vi "Ex3_Serial_Write_Read.vi"(0 "VISA resource":refnum<visa-resource-name>="COM4", 5 "Comando":T2(ring), 7 "Decisión":bool, 9 "stop":bool, 11 "error in (no error)":errorcluster) -> (3 "VISA resource 2":refnum<visa-resource-name>="COM4", 4 "Señales Digitales":dynamicdata(graph), 6 "Señales Analógicas":dynamicdata(graph), 8 "Buffer Filtrado":string, 10 "Cluster Señales":T1, 15 "error out":errorcluster)   [LabVIEW 2020]
uses:
  <vilib>/Instr/_visa.llb/VISA Configure Serial Port (Instr).vi
panel:
  out "Buffer Completo":string
  out "LISTO?":bool=TRUE
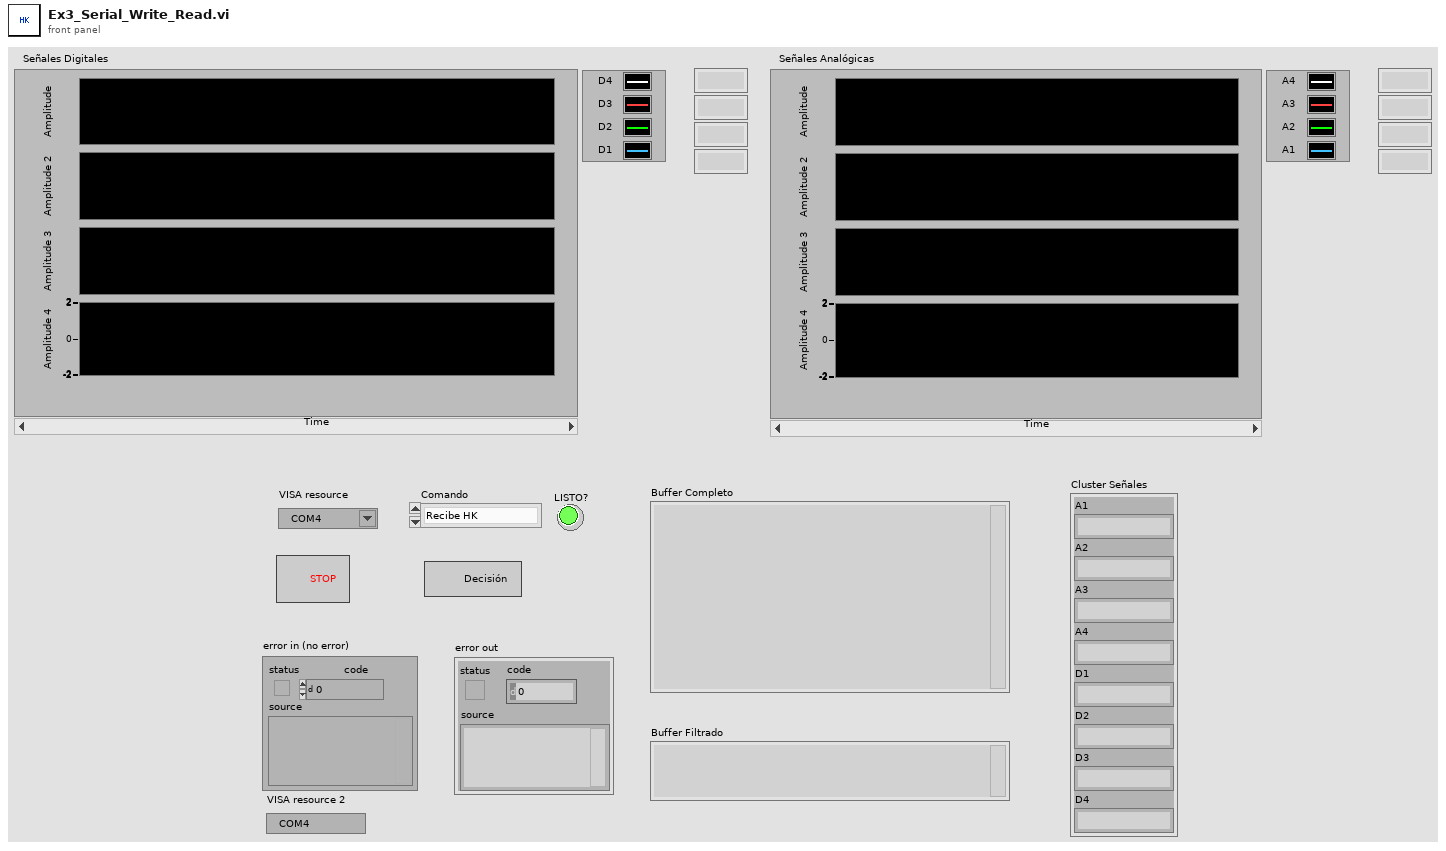
[diagram p1: front panel]
types:
  T1 = cluster{"A1":string, "A2":string, "A3":string, "A4":string, "D1":string, "D2":string, "D3":string, "D4":string}
  T2 = enum16{"Recibe HK", "Act Fecha", "Parametros", "Reset", "Stop"}
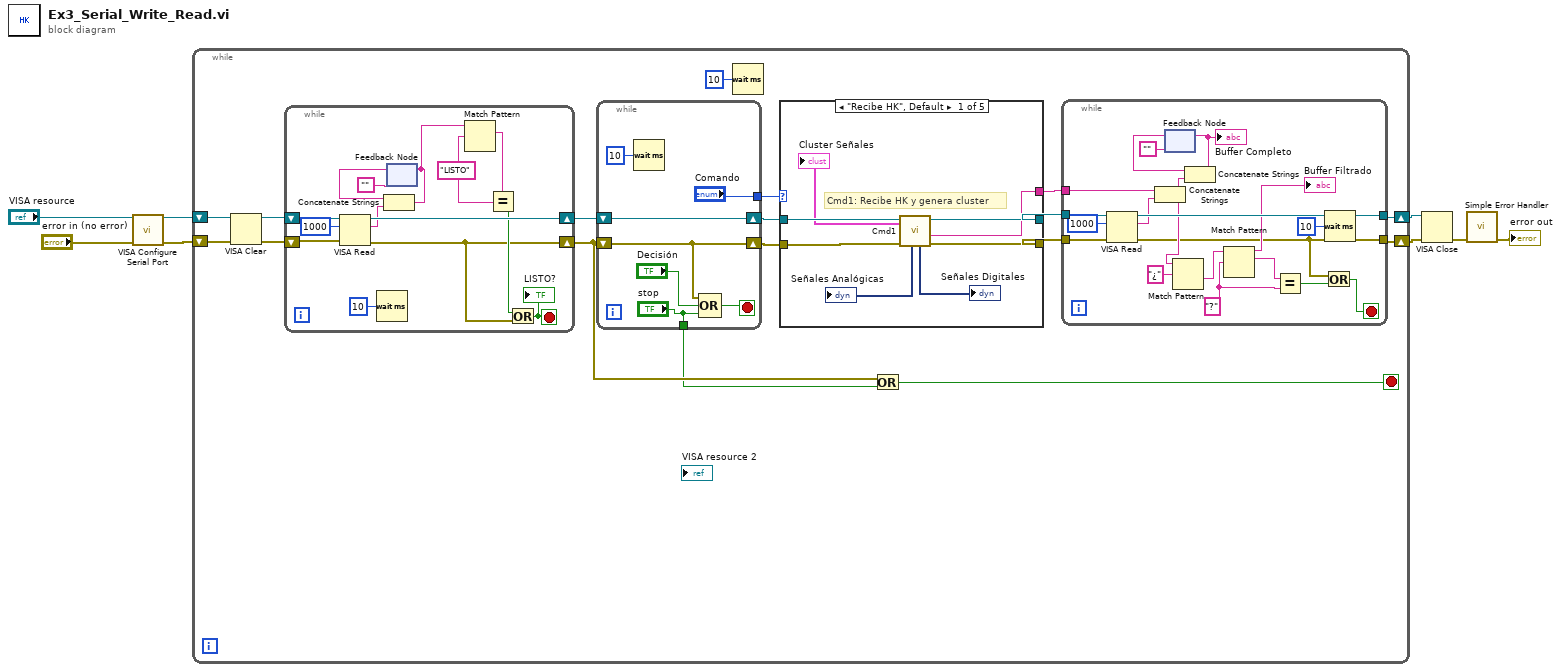
[diagram p0: block diagram]
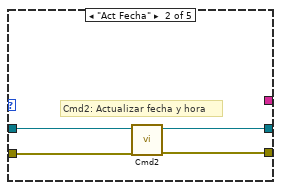
[diagram p2: hidden frame]
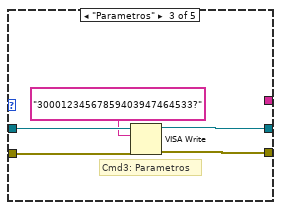
[diagram p3: hidden frame]
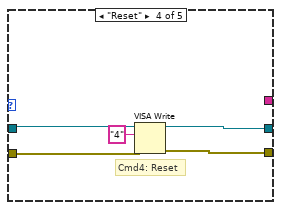
[diagram p4: hidden frame]
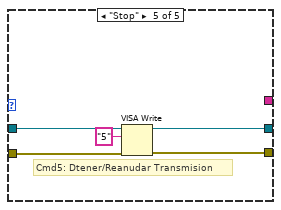
[diagram p5: hidden frame]
diagram:
  n1 = call-poly "VISA Configure Serial Port"("VISA resource name"="VISA resource", "error in (no error)"="error in (no error)") -> ("VISA resource name out"=w2:refnum<visa-resource-name>, "error out"=w1:errorcluster)  [unwired: 12 in]
  n2 = while {
    shift-right: [w12] -> w5
    shift-left: w1 -> [w18]
    shift-right: [w13] -> w6
    shift-left: w2 -> [w20]
    stop <- w21 stop-if-true
    n3 = VISA Clear(VISA resource name=w20, error in (no error)=w18) -> (VISA resource name out=w19:refnum<visa-resource-name>, error out=w17:errorcluster)
    n4 = while {
      shift-right: [w80] -> w11
      shift-left: w17 -> [w91]
      shift-right: [w89] -> w23
      shift-left: w19 -> [w92]
      stop <- w79 stop-if-true
      w82 = "LISTO" ("regular expression")
      n5 = VISA Read(VISA resource name=w92, byte count=u32 1000, error in (no error)=w91) -> (VISA resource name out=w89:refnum<visa-resource-name>, read buffer=w88:string, error out=w80:errorcluster)  [unwired: 1 out]
      n6 = Wait (ms)(milliseconds to wait=u32 10) -> ()  [unwired: 1 out]
      n7 = feedback #1("") -> (w87:string)
      n8 = Concatenate Strings(w87, w88) -> (w84:string)
      n9 = feedback-in #1(w84) -> ()
      n10 = Match Pattern(string=w84, regular expression=w82) -> (match substring=w83:string)  [unwired: 1 in, 3 out]
      n11 = Equal?(x=w83, y=w82) -> (x = y?=w81:bool)
      n12 = Or(x=w81, y=w80) -> (x .or. y?=w79:bool)
      "LISTO?" <- w79
    }
    n13 = while {
      tunnel: ["Comando"] -> w25
      shift-right: [w50] -> w24
      shift-left: w23 -> [w50]
      shift-right: [w47] -> w22
      shift-left: w11 -> [w47]
      tunnel: ["stop"] -> w10
      stop <- w48 stop-if-true
      n14 = Wait (ms)(milliseconds to wait=u32 10) -> ()  [unwired: 1 out]
      n15 = Compound Arithmetic op=OR(w47, "Decisión", "stop") -> (w48:bool)
    }
    n16 = Wait (ms)(milliseconds to wait=u32 10) -> ()  [unwired: 1 out]
    n17 = case shown="\"Recibe HK\", Default" w25 {
      tunnel: w24 -> [w59 w63 w66 w73 w78]
      tunnel: w22 -> [w58 w62 w65 w72 w76]
      tunnel: [w56 w61 w68 w70 w77] -> w15
      tunnel: [w57 w60 w67 w71 w75] -> w14
      tunnel: [w55 _ _ _ _] -> w9
      frame "Recibe HK", Default {
        # "Cmd1: Recibe HK y genera cluster"
        n18 = call "Cmd1.vi"("error in (no error)"=w58, "VISA Refnum in"=w59) -> ("error out (no error)"=w57:errorcluster, "read buffer"=w55:string, "VISA Refnum in 2"=w56:refnum<visa-resource-name>, "Señales Digitales"=→"Señales Digitales":dynamicdata, "Señales Analógicas"=→"Señales Analógicas":dynamicdata, "Señales"=→"Cluster Señales":T1)  [unwired: 4 in]
      }
      frame "Act Fecha" {
        # "Cmd2: Actualizar fecha y hora"
        n19 = call "Cmd2.vi"("error in (no error)"=w62, "VISA Refnum in"=w63) -> ("error out"=w60:errorcluster, "VISA Refnum out"=w61:refnum<visa-resource-name>)  [unwired: 7 in, 1 out]
      }
      frame "Parametros" {
        # "Cmd3: Parametros"
        n20 = VISA Write(VISA resource name=w66, write buffer="30001234567859403947464533?", error in (no error)=w65) -> (VISA resource name out=w68:refnum<visa-resource-name>, error out=w67:errorcluster)  [unwired: 1 out]
      }
      frame "Reset" {
        # "Cmd4: Reset"
        n21 = VISA Write(VISA resource name=w73, write buffer="4", error in (no error)=w72) -> (VISA resource name out=w70:refnum<visa-resource-name>, error out=w71:errorcluster)  [unwired: 1 out]
      }
      frame "Stop" {
        # "Cmd5: Dtener/Reanudar Transmision"
        n22 = VISA Write(VISA resource name=w78, write buffer="5", error in (no error)=w76) -> (VISA resource name out=w77:refnum<visa-resource-name>, error out=w75:errorcluster)  [unwired: 1 out]
      }
    }
    n23 = Or(x=w11, y=w10) -> (x .or. y?=w21:bool)
    n24 = while {
      tunnel: w15 -> [w42]
      tunnel: w14 -> [w41]
      tunnel: [w37] -> w13
      tunnel: [w27] -> w12
      tunnel: w9 -> [w29]
      stop <- w26 stop-if-true
      w38 = "?" ("regular expression")
      n25 = VISA Read(VISA resource name=w42, byte count=u32 1000, error in (no error)=w41) -> (VISA resource name out=w37:refnum<visa-resource-name>, read buffer=w34:string, error out=w27:errorcluster)  [unwired: 1 out]
      n26 = Concatenate Strings(w29, w34) -> (w33:string)
      n27 = feedback #2("") -> (w31:string)
      n28 = Match Pattern(string=w33, regular expression="¿") -> (after substring=w43:string)  [unwired: 1 in, 3 out]
      n29 = Concatenate Strings(w31, w33) -> (w32:string)
      "Buffer Completo" <- w32
      n30 = feedback-in #2(w32) -> ()
      n31 = Match Pattern(string=w43, regular expression=w38) -> (before substring=→"Buffer Filtrado":string, match substring=w36:string)  [unwired: 1 in, 2 out]
      n32 = Equal?(x=w36, y=w38) -> (x = y?=w28:bool)
      n33 = Or(x=w27, y=w28) -> (x .or. y?=w26:bool)
      n34 = Wait (ms)(milliseconds to wait=u32 10) -> ()  [unwired: 1 out]
    }
  }
  n35 = VISA Close(VISA resource name=w6, error in (no error)=w5) -> (error out=w8:errorcluster)
  n36 = call <vilib>:"Simple Error Handler.vi"("error in (no error)"=w8) -> ("error out"=→"error out":errorcluster)  [unwired: 4 in, 4 out]
